vi "gbtpFitModel.vi"(3 "output control":T1={"model function"=TRUE, "gradient"=FALSE}, 4 "data":variant, 5 "X":dbl[](array[numeric]), 6 "a":dbl[](array[numeric])) -> (0 "error out":errorcluster, 1 "f'(X,a)":dbl[](array[numeric]), 2 "f(X,a)":dbl[](array[numeric]))   [LabVIEW 2021]
uses:
  <vilib>/gmath/NumericalOptimization/LM_output select.ctl
  <vilib>/gmath/NI_Gmath.lvlib
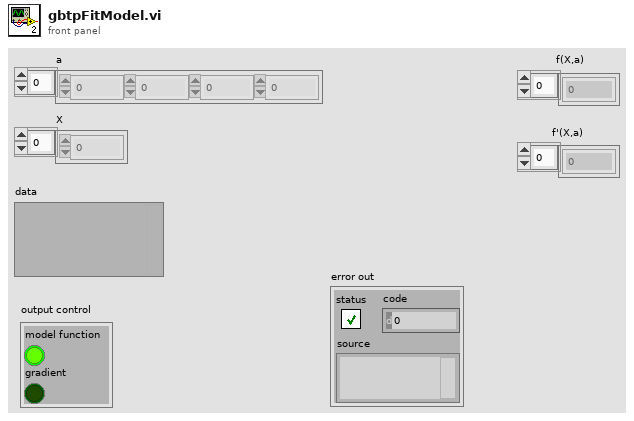
[diagram p1: front panel]
types:
  T1 = typedef "NI_Gmath.lvlib/LM_output select.ctl" = cluster{"model function":bool, "gradient":bool}
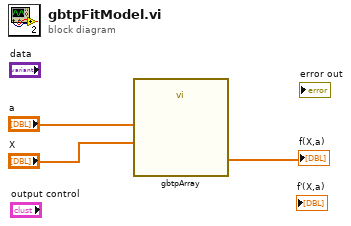
[diagram p0: block diagram]
diagram:
  n1 = call "gbtpArray.vi"("x"="X", "p"="a") -> ("f(x;p)"=→"f(X,a)":dbl[])  [unwired: 4 in]
